vi "close pcan.vi"(8 "error in (no error)":errorcluster, 11 "sock":i32) -> (0 "error out":errorcluster)   [LabVIEW 2024, in "libsocketcan_fd.lvlib"]
doc: "void close_pcan(int sock);"
uses:
  <userlib>/libsocketcan_fd/libsocketcan_fd.lvlib
  home/lvuser/natinst/bin/libsocketcan_fd.so
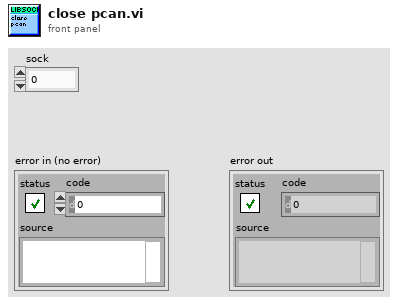
[diagram p1: front panel]
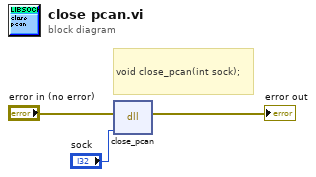
[diagram p0: block diagram]
diagram:
  # "void close_pcan(int sock);"
  n1 = dll-call lib="home/lvuser/natinst/bin/libsocketcan_fd.so" fn="close_pcan"(error in="error in (no error)", "sock"="sock") -> (error out=→"error out":errorcluster)  [unwired: 4 in, 1 out]
